vi "Load_from_Project.vi"(8 "error in (no error)":errorcluster, 9 "index":i32, 10 "buildObject":T3, 11 "AB_Container in":refnum<class "AB_Source_Container.lvclass">) -> (0 "error out":errorcluster, 2 "linker info":T2, 3 "AB_Container out":refnum<class "AB_Source_Container.lvclass">)   [LabVIEW 2020, in "AB_Source_Container.lvclass"]
uses:
  <vilib>/AppBuilder/AB_Classes/Source/Container/AB_Source_Container.lvclass
  <resource>/Framework/Providers/API/ItemRef.ctl
  <vilib>/Utility/lvfile.llb/LVFileType.ctl
  <vilib>/AppBuilder/RW_Project/AB_RW_Project_PropBag_Action.ctl
  <vilib>/AppBuilder/AB_Classes/Source/Container/AB_Source_Container.lvclass/AB_Source_Container.ctl
  <vilib>/AppBuilder/AB_Classes/Source/AB_Source.lvclass
  <vilib>/Utility/lvfile.llb/NI_FileType.lvlib
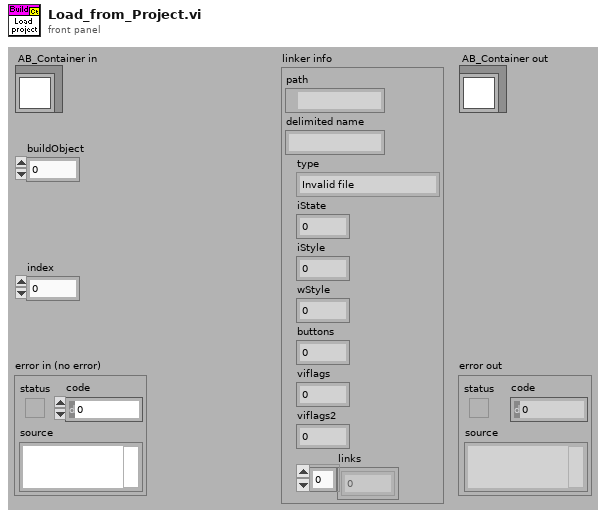
[diagram p1: front panel]
types:
  T1 = typedef "NI_FileType.lvlib/LVFileType.ctl" = enum32{"Invalid file", "Unknown type", "Instrument", "Control", "Polymorphic VI", "Project", "Library", "LVClass", "XControl", "XNode", "Shared library", ".NET assembly", "ActiveX interface", "CIN", "Run-time menu", "Palette menu", "Help file", "LLB", "XNode Edit Dependency", "Class Private Data Control", "Statechart", "MathScript .m file", "Ladder Diagram", "LVLibp", "XNode Build Dependency"}
  T2 = cluster{"path":path, "delimited name":string, "type":T1, "iState":u32, "iStyle":u16, "wStyle":u16, "buttons":u16, "viflags":u32, "viflags2":u32, "links":u32[]}
  T3 = typedef "ItemRef.ctl" = u64
  T4 = typedef "AB_RW_Project_PropBag_Action.ctl" = enum16{"read", "write", "clear", "readPrevious", "writePrevious", "clearPrevious"}
  T5 = typedef "AB_RW_Project_Source_Container_Data.ctl" = cluster{"applyInclusion":bool, "applyDestination":bool, "applyProperties":bool, "applyPassword":bool, "applyPrefix":bool, "applySaveSetttings":bool, "dependentDestinationIndex":i32}
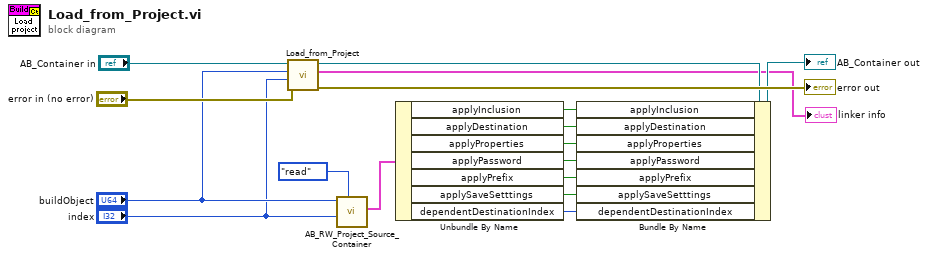
[diagram p0: block diagram]
diagram:
  n1 = call-parent "Load_from_Project.vi"("error in (no error)"="error in (no error)", "index"="index", "buildObject"="buildObject", "AB_Source in"="AB_Container in") -> ("error out"=→"error out":errorcluster, "linker info"=→"linker info":T2, "AB_Source out"=w14:refnum<class "AB_Source_Container.lvclass">)  [unwired: 5 out]
  n2 = call <vilib>:"AB_RW_Project_Source_Container.vi"("action"=AB_RW_Project_PropBag_Action."read", "index in"="index", "buildObject"="buildObject") -> ("dataSource out"=w9:T5)  [unwired: 2 in, 6 out]
  n3 = Unbundle By Name(w9) -> ("applyInclusion"=w8:bool, "applyDestination"=w7:bool, "applyProperties"=w6:bool, "applyPassword"=w5:bool, "applyPrefix"=w4:bool, "applySaveSetttings"=w3:bool, "dependentDestinationIndex"=w1:i32)
  n4 = Bundle By Name(cluster=w14, "applyInclusion"=w8, "applyDestination"=w7, "applyProperties"=w6, "applyPassword"=w5, "applyPrefix"=w4, "applySaveSetttings"=w3, "dependentDestinationIndex"=w1) -> (→"AB_Container out":refnum<class "AB_Source_Container.lvclass">)
